vi "WriteParametersToXML.vi"(0 "GenerateInteropAssembly":T4, 1 "SetVIInformationArray":T2[](array[typedef]), 2 "SetLVCLassInformationArray":T3[](array[typedef]), 3 "GenAssemblyConstructor":T1, 4 "XMLParam":path=path "c:/constructor.xml") -> ()   [LabVIEW 2020]
uses:
  <vilib>/Utility/xml.llb/Write to XML File(string).vi
  <vilib>/AppBuilder/AB_InteropAssembly_GenerateInteropAssembly_Info.ctl
  <vilib>/AppBuilder/AB_InteropAssembly_SetLVClassInformation.ctl
  <vilib>/AppBuilder/AB_InteropAssembly_SetVIInformation.ctl
  <vilib>/AppBuilder/AB_InteropAssembly_GenAssemblyConstructor_Info.ctl
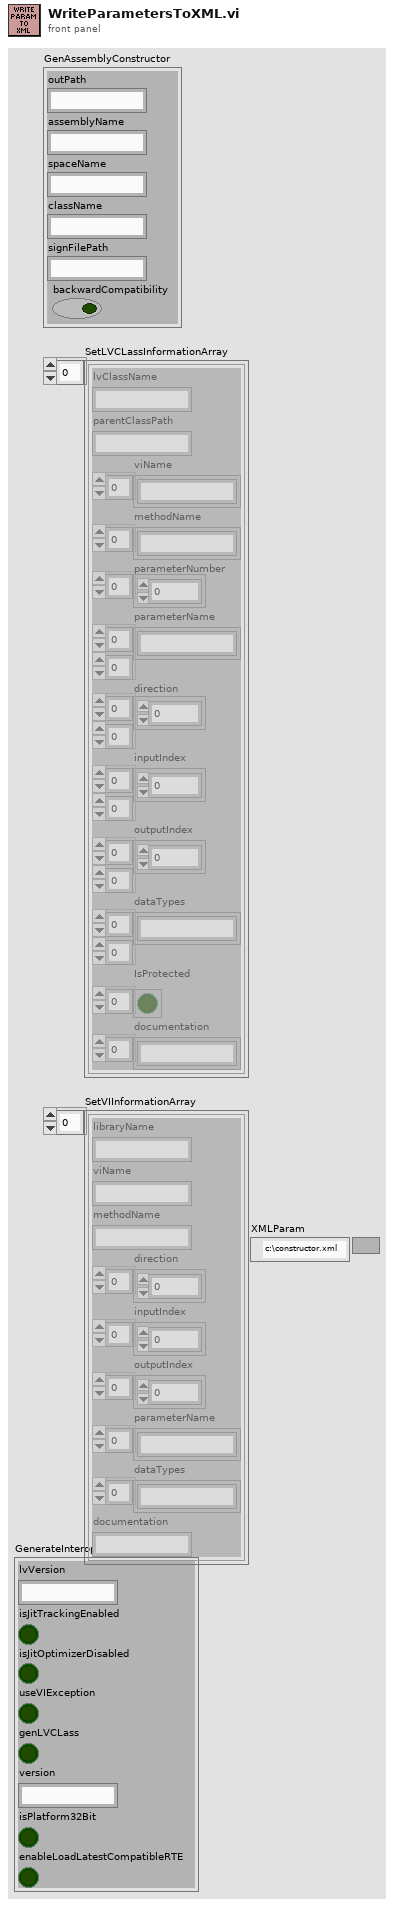
[diagram p1: front panel]
types:
  T1 = typedef "AB_InteropAssembly_GenAssemblyConstructor_Info.ctl" = cluster{"outPath":string, "assemblyName":string, "spaceName":string, "className":string, "signFilePath":string, "backwardCompatibility":bool}
  T2 = typedef "AB_InteropAssembly_SetVIInformation.ctl" = cluster{"libraryName":string, "viName":string, "methodName":string, "direction":i32[], "inputIndex":i32[], "outputIndex":i32[], "parameterName":string[], "dataTypes":string[], "documentation":string}
  T3 = typedef "AB_InteropAssembly_SetLVClassInformation.ctl" = cluster{"lvClassName":string, "parentClassPath":string, "viName":string[], "methodName":string[], "parameterNumber":i32[], "parameterName":string[][], "direction":i32[][], "inputIndex":i32[][], "outputIndex":i32[][], "dataTypes":string[][], "IsProtected":bool[], "documentation":string[]}
  T4 = typedef "AB_InteropAssembly_GenerateInteropAssembly_Info.ctl" = cluster{"lvVersion":string, "isJitTrackingEnabled":bool, "isJitOptimizerDisabled":bool, "useVIException":bool, "genLVCLass":bool, "version":string, "isPlatform32Bit":bool, "enableLoadLatestCompatibleRTE":bool}
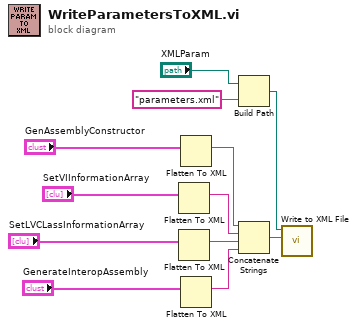
[diagram p0: block diagram]
diagram:
  n1 = Flatten To XML(6:"SetVIInformationArray") -> (2:w9:string)
  n2 = Flatten To XML(6:"SetLVCLassInformationArray") -> (2:w10:string)
  n3 = Flatten To XML(6:"GenAssemblyConstructor") -> (2:w8:string)
  n4 = Flatten To XML(6:"GenerateInteropAssembly") -> (2:w11:string)
  n5 = Build Path(base path="XMLParam", name or relative path="parameters.xml") -> (appended path=w1:path)
  n6 = Concatenate Strings(w8, w9, w10, w11) -> (w12:string)
  n7 = call-poly <vilib>:"Write to XML File.vi"("XML Input"=w12, "XML File Path"=w1) -> ()  [unwired: 7 in, 3 out]
